vi "Copia_fichero_a_directorio.vi"(8 "error in (no error)":errorcluster, 10 "source path":path, 11 "Target path":path) -> (0 "error out":errorcluster, 3 "new path":path)   [LabVIEW 2019]
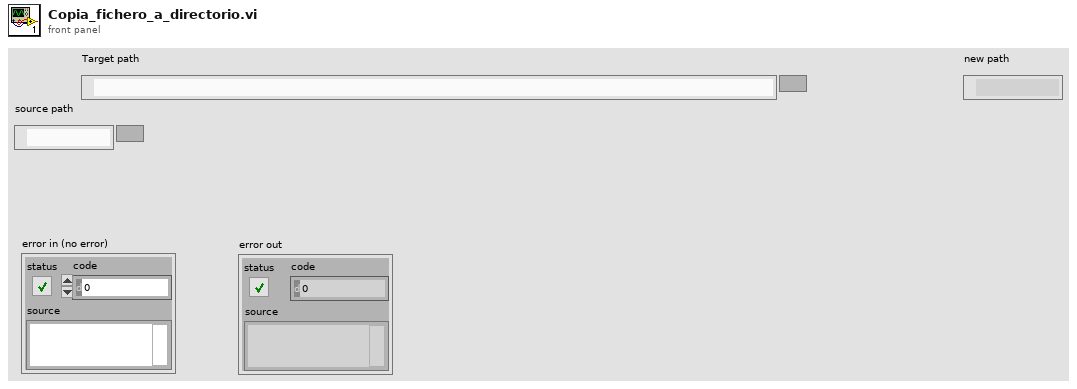
[diagram p1: front panel]
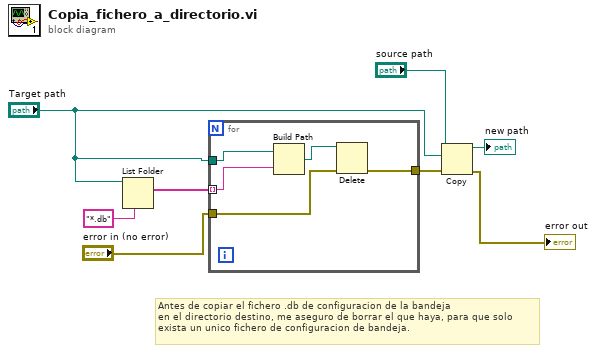
[diagram p0: block diagram]
diagram:
  # "Antes de copiar el fichero .db de configuracion de la bandeja\nen el directorio destino, me aseguro de borrar el que haya, para que solo\nexista un unico fichero de configuracion de bandeja."
  n1 = List Folder(path="Target path", pattern="*.db") -> (filenames=w7:string[])  [unwired: 2 in, 3 out]
  n2 = for {
    tunnel: w7 -> [w12] mode=indexing
    tunnel: "Target path" -> [w13]
    tunnel: "error in (no error)" -> [w10]
    tunnel: [w9] -> w3
    n3 = Build Path(base path=w13, name or relative path=w12) -> (appended path=w11:path)
    n4 = Delete(path (use dialog)=w11, error in=w10) -> (error out=w9:errorcluster)  [unwired: 3 in, 2 out]
  }
  n5 = Copy(8:w3, 10:"Target path", 11:"source path") -> (0:→"error out":errorcluster, 3:→"new path":path)  [unwired: 2 in, 1 out]
